vi "Master Table Config File - Update Node.vi"(8 "error in (no error)":errorcluster, 10 "Local Channels Table Size In":u64, 11 "Compiled.Settings In":T1) -> (0 "error out":errorcluster, 3 "Compiled.Settings Out":T1)   [LabVIEW 2016, in "PXImc Custom Device System Explorer.lvlib"]
uses:
  PXImc Custom Device System Explorer.lvlib
  Shared/Compiled.Settings.ctl
  PXImc Router/Controls/Target Type.ctl
  PXImc Router/Controls/Router - Configuration.ctl
  PXImc Router/Controls/Router/Node Block R-W Properties.ctl
  PXImc Router/Controls/Router/Block Properties.ctl
  PXImc Router/Controls/Router/Router - PXImc Properties.ctl
  PXImc Router/Controls/Router/Router - PXImc Card Properties.ctl
  PXImc Router/Controls/Node Data.ctl
  PXImc Router/Controls/Node/Node - PXImc Parameters.ctl
  PXImc Router/Controls/Node/Node - Writer Data.ctl
  PXImc Router/Controls/Node/Node Ch Properties.ctl
  PXImc Router/Controls/Data Type.ctl
  PXImc Router/Controls/Node/Node - Readers Data.ctl
  PXImc Router/Controls/Node/Node - Reader Data.ctl
  <vilib>/Utility/file.llb/Read Delimited Spreadsheet (string).vi
  <vilib>/Utility/file.llb/Write Delimited Spreadsheet (string).vi
  PXImc Router/PXImc Router.lvlib
  Shared/PXImc Custom Device Shared.lvlib
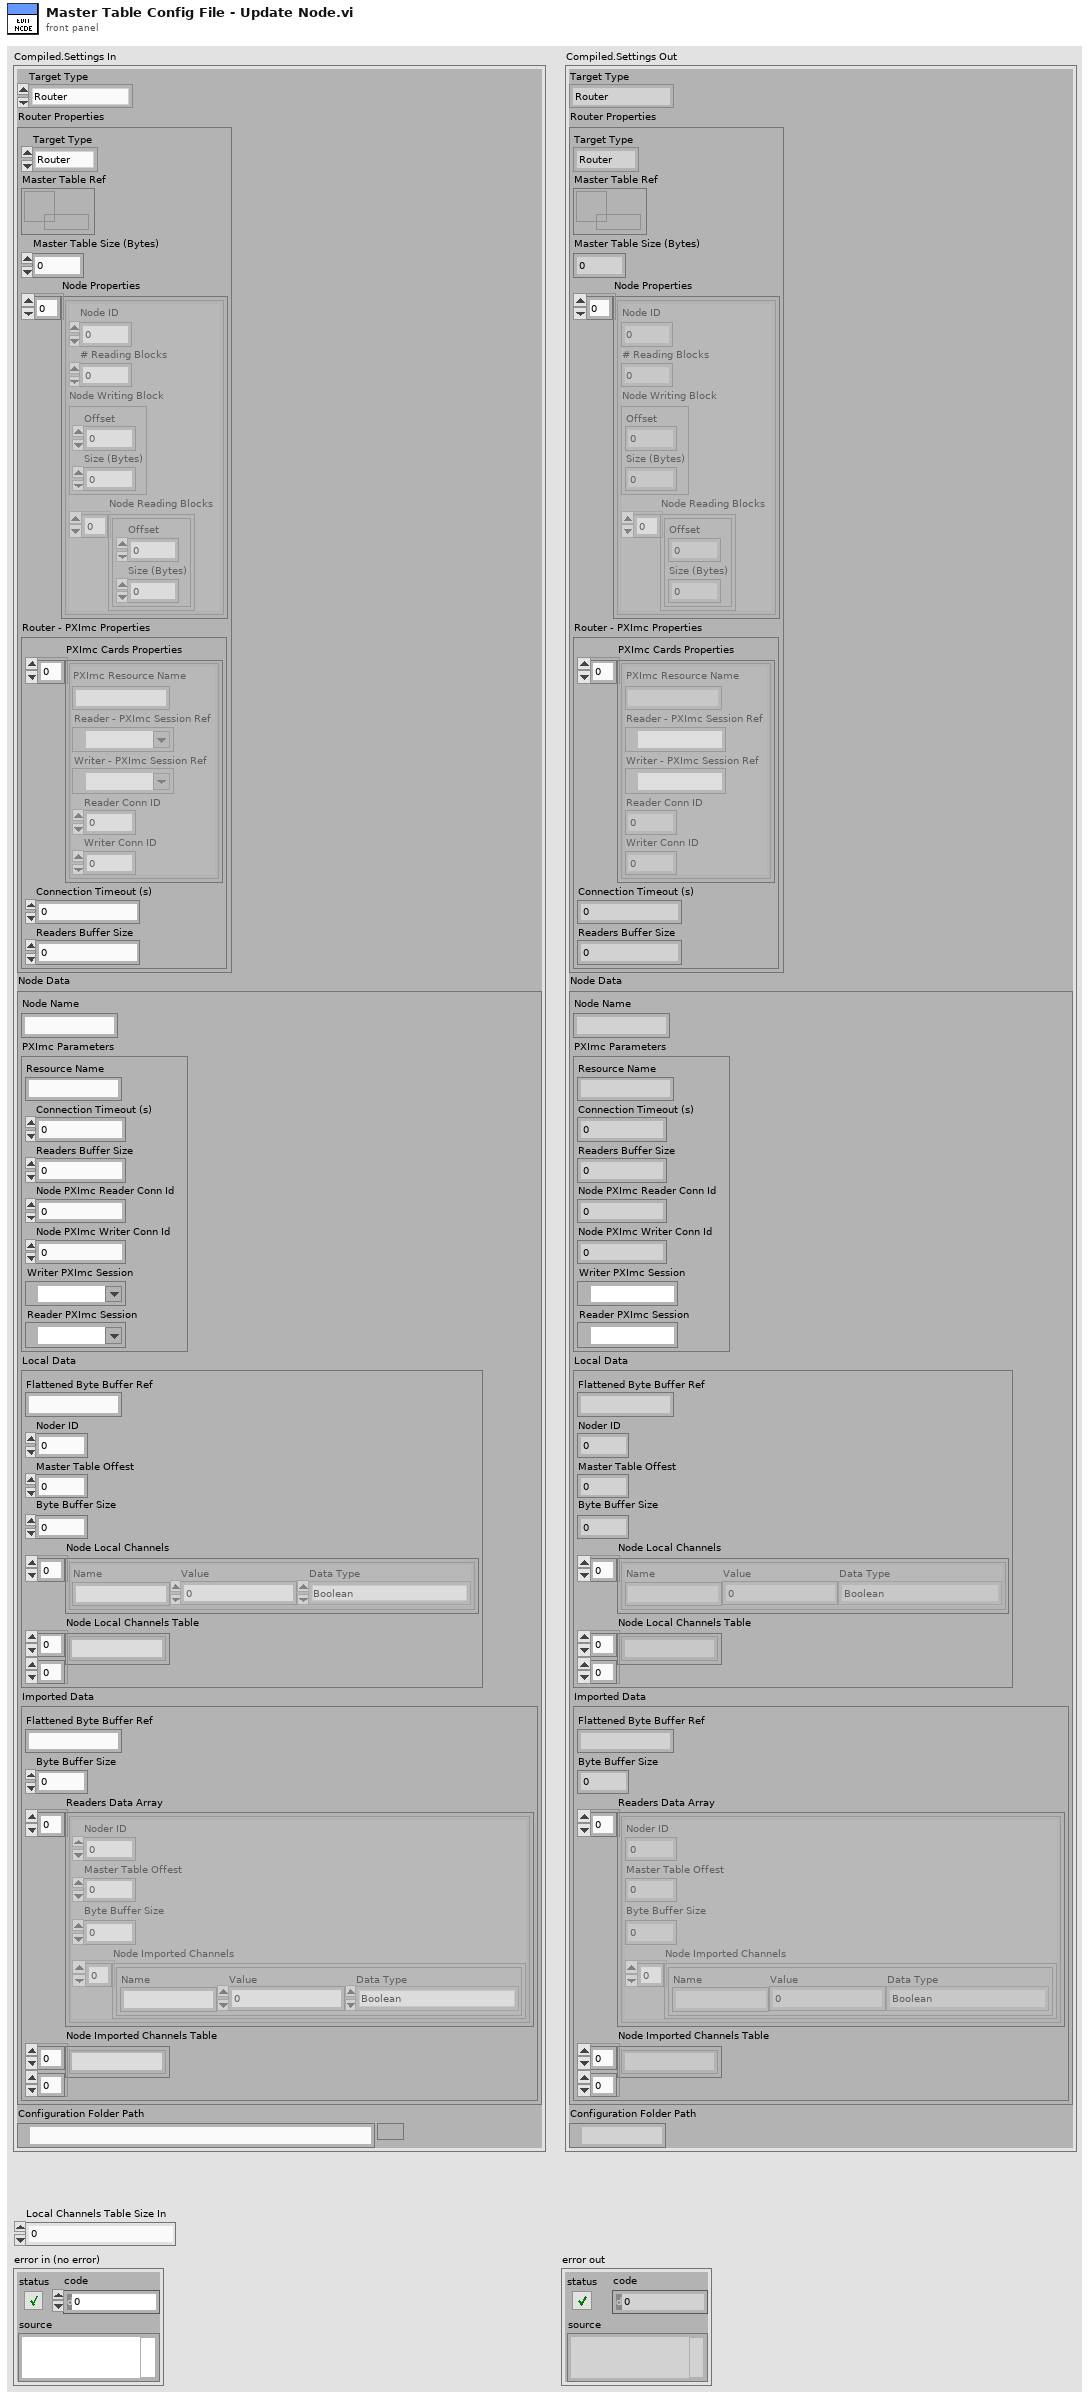
[diagram p1: front panel]
types:
  T1 = typedef "PXImc Custom Device Shared.lvlib/Compiled.Settings.ctl" = cluster{"Target Type":T2, "Router Properties":T3, "Node Data":T8, "Configuration Folder Path":path}
  T2 = typedef "PXImc Router.lvlib/Target Type.ctl" = enum16{"Router", "Node"}
  T3 = typedef "PXImc Router.lvlib/Router - Configuration.ctl" = cluster{"Target Type":T2, "Master Table Ref":refnum<data-value>, "Master Table Size (Bytes)":u32, "Node Properties":T4[], "Router - PXImc Properties":T6}
  T4 = typedef "PXImc Router.lvlib/Node Block R-W Properties.ctl" = cluster{"Node ID":u32, "# Reading Blocks":u32, "Node Writing Block":T5, "Node Reading Blocks":T5[]}
  T5 = typedef "PXImc Router.lvlib/Block Properties.ctl" = cluster{"Offset":u32, "Size (Bytes)":u32}
  T6 = typedef "PXImc Router.lvlib/Router - PXImc Properties.ctl" = cluster{"PXImc Cards Properties":T7[], "Connection Timeout (s)":dbl, "Readers Buffer Size":u64}
  T7 = typedef "PXImc Router.lvlib/Router - PXImc Card Properties.ctl" = cluster{"PXImc Resource Name":string, "Reader - PXImc Session Ref":refnum<k21>, "Writer - PXImc Session Ref":refnum<k21>, "Reader Conn ID":u16, "Writer Conn ID":u16}
  T8 = typedef "PXImc Router.lvlib/Node Data.ctl" = cluster{"Node Name":string, "PXImc Parameters":T9, "Local Data":T10, "Imported Data":T13}
  T9 = typedef "PXImc Router.lvlib/Node - PXImc Parameters.ctl" = cluster{"Resource Name":string, "Connection Timeout (s)":dbl, "Readers Buffer Size":u64, "Node PXImc Reader Conn Id":u16, "Node PXImc Writer Conn Id":u16, "Writer PXImc Session":refnum<k21>, "Reader PXImc Session":refnum<k21>}
  T10 = typedef "PXImc Router.lvlib/Node - Writer Data.ctl" = cluster{"Flattened Byte Buffer Ref":string, "Noder ID":u32, "Master Table Offest":u32, "Byte Buffer Size":u32, "Node Local Channels":T11[], "Node Local Channels Table":string[][]}
  T11 = typedef "PXImc Router.lvlib/Node Ch Properties.ctl" = cluster{"Name":string, "Value":dbl, "Data Type":T12}
  T12 = typedef "PXImc Router.lvlib/Data Type.ctl" = enum16{"Boolean", "SGL", "DBL", "I8", "I16", "I32", "I64", "U8", "U16", "U32", "U64"}
  T13 = typedef "PXImc Router.lvlib/Node - Readers Data.ctl" = cluster{"Flattened Byte Buffer Ref":string, "Byte Buffer Size":u64, "Readers Data Array":T14[], "Node Imported Channels Table":string[][]}
  T14 = typedef "PXImc Router.lvlib/Node - Reader Data.ctl" = cluster{"Noder ID":u32, "Master Table Offest":u32, "Byte Buffer Size":u64, "Node Imported Channels":T11[]}
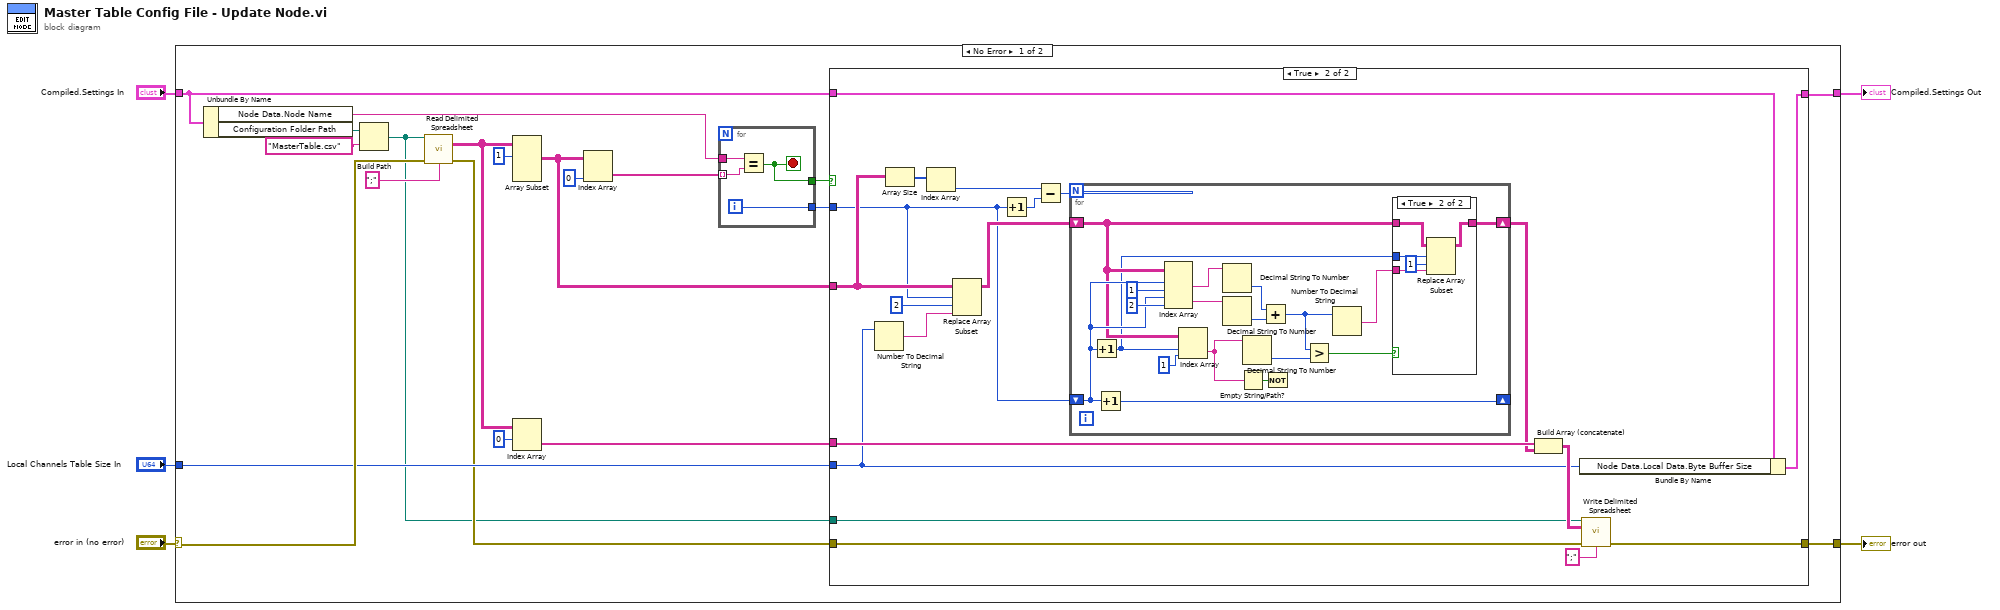
[diagram p0: block diagram]
diagram:
  n1 = case shown="No Error" "error in (no error)" {
    selector: "error in (no error)" -> [w24 w76]
    tunnel: [w10 w76] -> w4
    tunnel: "Compiled.Settings In" -> [w9 w75]
    tunnel: [w8 w75] -> w2
    tunnel: "Local Channels Table Size In" -> [w12 _]
    frame No Error {
      n2 = Unbundle By Name(w9) -> ("Node Data.Node Name"=w6:string, "Configuration Folder Path"=w23:path)
      n3 = Build Path(base path=w23, name or relative path="MasterTable.csv") -> (appended path=w7:path)
      n4 = call-poly <vilib>:"Read Delimited Spreadsheet.vi"("file path (dialog if empty)"=w7, "error in (no error)"=w24, "delimiter (\\t)"=";" ("delimiter (\\t)")) -> ("all rows"=w20:string[][], "error out"=w11:errorcluster)  [unwired: 7 in, 4 out]
      n5 = Array Subset(array=w20, index (row)=1 ("index")) -> (w15:string[][])  [unwired: 3 in]
      n6 = Index Array(array=w20, index (row)=0) -> (element=w13:string[])  [unwired: 1 in]
      n7 = Index Array(array=w15, index (col)=0 ("disabled index (col)")) -> (element=w17:string[])  [unwired: 1 in]
      n8 = for {
        tunnel: w17 -> [w28] mode=indexing
        tunnel: w6 -> [w29]
        tunnel: [w27] -> w16
        tunnel: [w26] -> w14
        i -> [w26]
        stop <- w27 stop-if-true
        n9 = Equal?(x=w29, y=w28) -> (x = y?=w27:bool)
      }
      n10 = case shown="True" w16 {
        tunnel: w15 -> [_ w38]
        tunnel: w14 -> [_ w32]
        tunnel: w13 -> [_ w45]
        tunnel: w12 -> [_ w40]
        tunnel: w11 -> [w30 w47]
        tunnel: [w30 w46] -> w10
        tunnel: w9 -> [w31 w44]
        tunnel: [w31 w43] -> w8
        tunnel: w7 -> [_ w42]
        frame False {
        }
        frame True {
          n11 = Number To Decimal String(number=w40) -> (decimal integer string=w50:string)  [unwired: 1 in]
          n12 = Array Size(array=w38) -> (size(s)=w37:i32[])
          n13 = Index Array(array=w37) -> (element=w36:i32)  [unwired: 1 in]
          n14 = Replace Array Subset(array=w38, new element=w50, index (row)=w32, index (col)=2 ("disabled index (col)")) -> (w39:string[][])
          n15 = Increment(x=w32) -> (x+1=w35:i32)
          n16 = Subtract(x=w36, y=w35) -> (x-y=w34:i32)
          n17 = for {
            N: w34 -> [_]
            shift-right: [w57] -> _
            shift-left: w32 -> [w58]
            shift-right: [w51] -> w33
            shift-left: w39 -> [w56]
            n18 = Increment(x=w58) -> (x+1=w55:i32)
            n19 = Increment(x=w58) -> (x+1=w57:i32)
            n20 = Index Array(array=w56, index (row) #1=w58, index (col) #1=1 ("disabled index (col)"), index (row) #2=w58, index (col) #2=2 ("disabled index (col)")) -> (element #1=w66:string, element #2=w61:string)
            n21 = Index Array(array=w56, index (row)=w55, index (col)=1 ("disabled index (col)")) -> (element=w64:string)
            n22 = Decimal String To Number(string=w66) -> (number=w60:i32)  [unwired: 2 in, 1 out]
            n23 = Decimal String To Number(string=w61) -> (number=w59:i32)  [unwired: 2 in, 1 out]
            n24 = Empty String/Path?(string/path=w64) -> (empty?=w67:bool)
            n25 = Decimal String To Number(string=w64) -> (number=w68:i32)  [unwired: 2 in, 1 out]
            n26 = Add(x=w60, y=w59) -> (x+y=w53:i32)
            n27 = Not(x=w67) -> ()  [unwired: 1 out]
            n28 = Greater?(x=w53, y=w68) -> (0:w54:bool)
            n29 = Number To Decimal String(number=w53) -> (decimal integer string=w52:string)  [unwired: 1 in]
            n30 = case shown="True" w54 {
              tunnel: w56 -> [w69 w74]
              tunnel: w55 -> [_ w72]
              tunnel: w52 -> [_ w71]
              tunnel: [w69 w70] -> w51
              frame False {
              }
              frame True {
                n31 = Replace Array Subset(array=w74, new element=w71, index (row)=w72, index (col)=1 ("disabled index (col)")) -> (w70:string[][])
              }
            }
          }
          n32 = Build Array (concatenate)(w45, w33) -> (w49:string[][])
          n33 = Bundle By Name(cluster=w44, "Node Data.Local Data.Byte Buffer Size"=w40) -> (w43:T1)
          n34 = call-poly <vilib>:"Write Delimited Spreadsheet.vi"("file path (dialog if empty)"=w42, "2D data"=w49, "error in (no error)"=w47, "delimiter (\\t)"=";" ("delimiter (\\t)")) -> ("error out"=w46:errorcluster)  [unwired: 10 in, 1 out]
        }
      }
    }
    frame Error {
    }
  }
  "error out" <- w4
  "Compiled.Settings Out" <- w2
